vi "Colors Separator.vi"(8 "error in (no error)":errorcluster, 10 "Boolean":bool, 11 "TbCntr in":refnum<class "TabControl.lvclass">) -> (0 "error out":errorcluster, 3 "TbCntr out":refnum<class "TabControl.lvclass">)   [LabVIEW 2020, in "TabControl.lvclass"]
uses:
  TabControl.lvclass
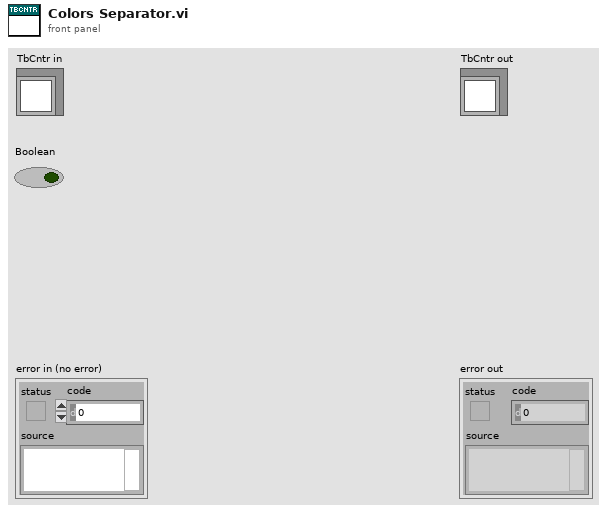
[diagram p1: front panel]
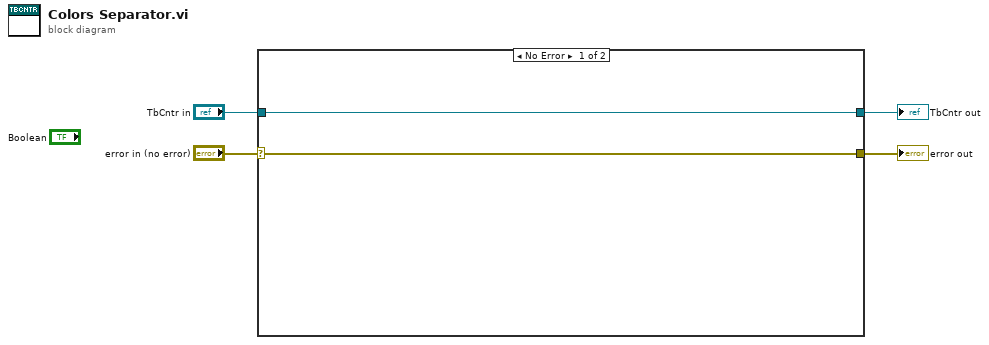
[diagram p0: block diagram]
diagram:
  n1 = case shown="No Error" "error in (no error)" {
    selector: "error in (no error)" -> [w5 w8]
    tunnel: [w5 w8] -> w3
    tunnel: [w6 w7] -> w1
    tunnel: "TbCntr in" -> [w6 w7]
    frame No Error {
    }
    frame Error {
    }
  }
  "error out" <- w3
  "TbCntr out" <- w1
